vi "FTW-Endpoint-CreateRequester.vi"(0 "FTW Endpoint":refnum<class "FTW-Endpoint-TCP.lvclass">, 5 "Endpoint Address":string, 11 "error in":errorcluster) -> (4 "FTW Endpoint out":refnum<class "FTW-Endpoint-TCP.lvclass">, 15 "error out":errorcluster)   [LabVIEW 2013, in "FTW-Endpoint-TCP.lvclass"]
uses:
  FTW-Endpoint-TCP.lvclass
panel:
  # "Inputs"
  # "Outputs"
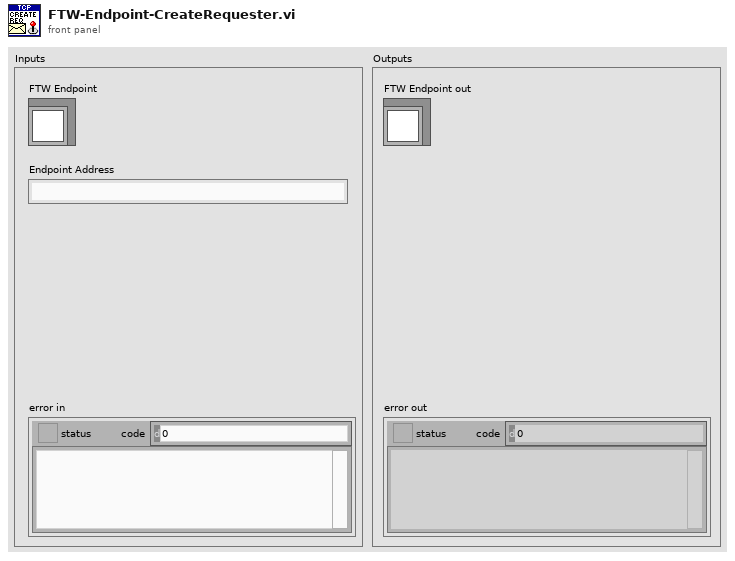
[diagram p1: front panel]
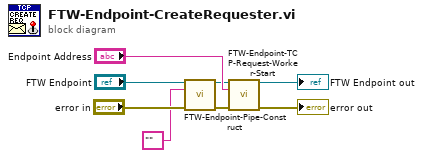
[diagram p0: block diagram]
diagram:
  n1 = call-dynamic "FTW-Endpoint-Pipe-Construct.vi"("FTW Endpoint"="FTW Endpoint", "Address"="" ("empty string"), "error in"="error in") -> ("FTW Endpoint out"=w2:refnum<class "FTW-Endpoint-TCP.lvclass">, "error out"=w3:errorcluster)  [unwired: 10 in, 1 out]
  n2 = call-dynamic "FTW-Endpoint-TCP-Request-Worker-Start.vi"("FTW-Endpoint-TCP In"=w2, "Endpoint Address"="Endpoint Address", "error in"=w3) -> ("FTW-Endpoint-TCP Out"=→"FTW Endpoint out":refnum<class "FTW-Endpoint-TCP.lvclass">, "error out"=→"error out":errorcluster)  [unwired: 11 in]
